vi "Decode HydroHarp v2 TT Data.vi"(8 "oflcorr_in":u64, 11 "rawbits":u32) -> (0 "oflcorr_out":u64, 1 "channel":u8, 3 "truetime":u64, 4 "markercode":u32)   [LabVIEW 2021, in "PTU Files.lvlib"]
uses:
  PTU Files.lvlib
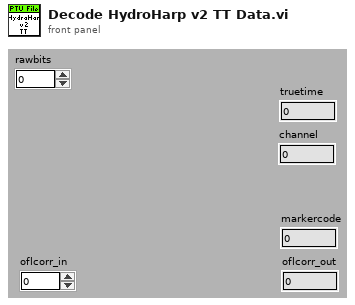
[diagram p1: front panel]
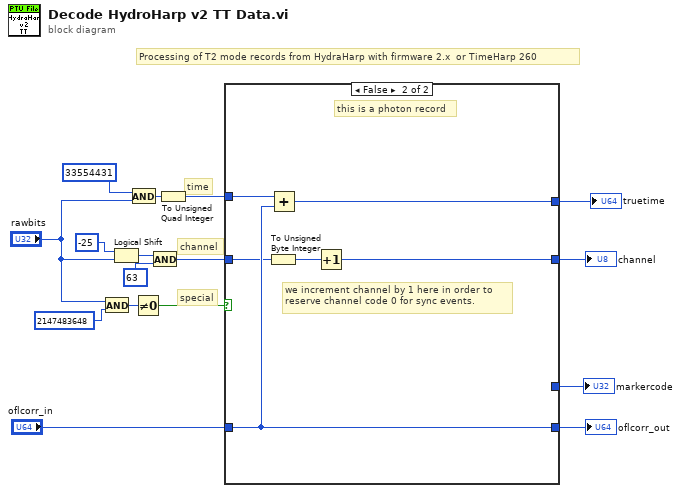
[diagram p0: block diagram]
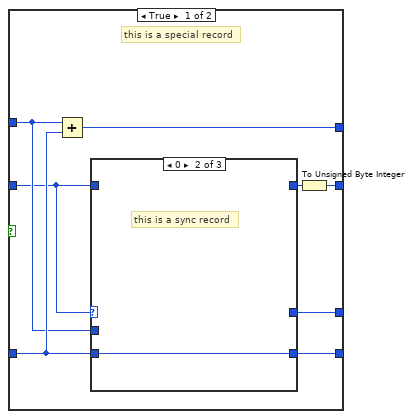
[diagram p2: hidden frame]
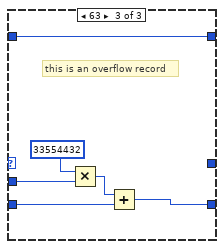
[diagram p4: hidden frame]
diagram:
  # "special"
  # "Processing of T2 mode records from HydraHarp with firmware 2.x  or TimeHarp 260"
  # "channel"
  # "time"
  n1 = And(x="rawbits", y=u32 2147483648 ("x")) -> (x .and. y?=w4:u32)
  n2 = Logical Shift(y=-25, x="rawbits") -> (x << y=w12:u32)
  n3 = And(x=u32 33554431, y="rawbits") -> (x .and. y?=w8:u32)
  n4 = Not Equal To 0?(x=w4) -> (x != 0?=w3:bool)
  n5 = And(x=w12, y=u32 63 ("x")) -> (x .and. y?=w15:u32)
  n6 = To Unsigned Quad Integer(1:w8) -> (0:w1:u64)
  n7 = case shown="False" w3 {
    tunnel: w1 -> [w20 w39]
    tunnel: "oflcorr_in" -> [w22 w37]
    tunnel: [w24 w37] -> w10
    tunnel: [w23 _] -> w11
    tunnel: [w21 w38] -> w14
    tunnel: [w17 w35] -> w16
    tunnel: w15 -> [w19 w36]
    frame True {
      # "this is a special record"
      n8 = Add(x=w20, y=w22) -> (x+y=w21:u64)
      n9 = case shown="0" w19 {
        selector: w19 -> [w25 _ _]
        tunnel: w22 -> [w26 w27 w33]
        tunnel: [w26 w27 w32] -> w24
        tunnel: [w25 _ _] -> w23
        tunnel: w20 -> [_ _ w30]
        tunnel: w19 -> [_ _ w28]
        tunnel: [_ _ w28] -> w18
        frame Default {
          # "this is a marker record"
        }
        frame 0 {
          # "this is a sync record"
        }
        frame 63 {
          # "this is an overflow record"
          n10 = Multiply(x=u64 33554432, y=w30) -> (x*y=w29:u64)
          n11 = Add(x=w29, y=w33) -> (x+y=w32:u64)
        }
      }
      n12 = To Unsigned Byte Integer(number=w18) -> (unsigned 8bit integer=w17:u8)
    }
    frame False {
      # "we increment channel by 1 here in order to\nreserve channel code 0 for sync events."
      # "this is a photon record"
      n13 = To Unsigned Byte Integer(number=w36) -> (unsigned 8bit integer=w34:u8)
      n14 = Add(x=w39, y=w37) -> (x+y=w38:u64)
      n15 = Increment(x=w34) -> (x+1=w35:u8)
    }
  }
  "channel" <- w16
  "truetime" <- w14
  "markercode" <- w11
  "oflcorr_out" <- w10
